vi "find closest point.vi"(11 "Path Data":T1={"Path"=[], "Target Velocities"=[], "Robot Location"=[], "Relative Robot Angle (rad)"=0.0, "Curvature"=0.0, "Lookahead Point"=[3064.399009129367, 18229.833030071386], "Lookahead Index"=8.422809037111724, "Closest Point"=[], "Closest Point Index"=0, "Left Velocity"=0.0, "Right Velocity"=0.0, "Left Encoder Vel"=0, "Right Encoder Vel"=0, "Left Encoder Pos"=0, "Right Encoder Pos"=0, "Inital Robot Angle (deg)"=0.0}) -> (3 "Path Data":T1={"Path"=[], "Target Velocities"=[], "Robot Location"=[], "Relative Robot Angle (rad)"=0.0, "Curvature"=0.0, "Lookahead Point"=[3064.399009129367, 18229.833030071386], "Lookahead Index"=8.422809037111724, "Closest Point"=[], "Closest Point Index"=0, "Left Velocity"=0.0, "Right Velocity"=0.0, "Left Encoder Vel"=0, "Right Encoder Vel"=0, "Left Encoder Pos"=0, "Right Encoder Pos"=0, "Inital Robot Angle (deg)"=0.0})   [LabVIEW 2018]
uses:
  path data.ctl
panel:
  out "Closest Point Index":i32
  out "Closest Point":dbl[](array[numeric])
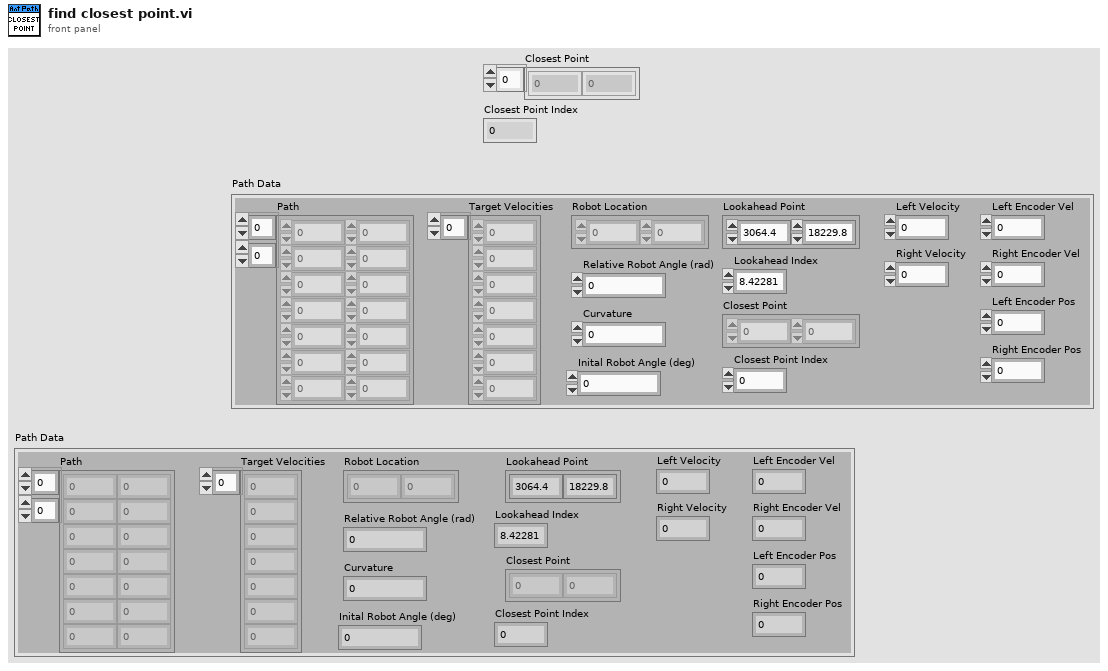
[diagram p1: front panel]
types:
  T1 = typedef "path data.ctl" = cluster{"Path":dbl[][], "Target Velocities":dbl[], "Robot Location":dbl[], "Relative Robot Angle (rad)":dbl, "Curvature":dbl, "Lookahead Point":dbl[], "Lookahead Index":dbl, "Closest Point":dbl[], "Closest Point Index":i32, "Left Velocity":dbl, "Right Velocity":dbl, "Left Encoder Vel":i32, "Right Encoder Vel":i32, "Left Encoder Pos":i32, "Right Encoder Pos":i32, "Inital Robot Angle (deg)":dbl}
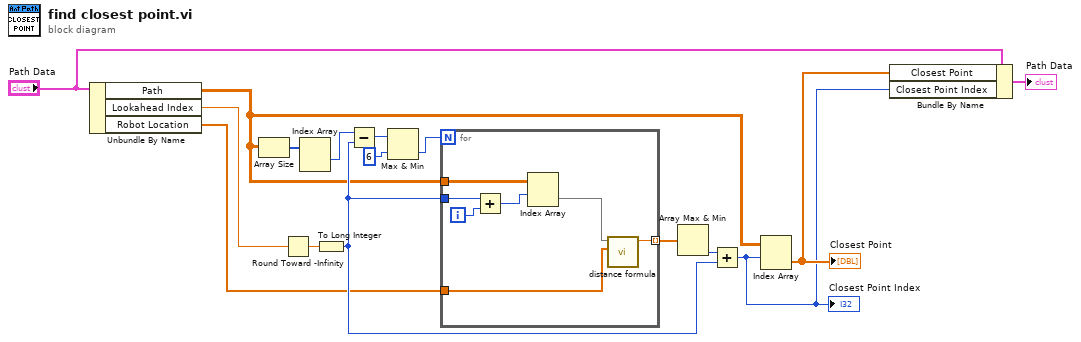
[diagram p0: block diagram]
diagram:
  n1 = Unbundle By Name("Path Data") -> ("Path"=w3:dbl[][], "Lookahead Index"=w2:dbl, "Robot Location"=w1:dbl[])
  n2 = Array Size(array=w3) -> (size(s)=w16:i32[])
  n3 = Round Toward -Infinity(1:w2) -> (0:w14:dbl)
  n4 = Index Array(array=w16) -> (element #1=w15:i32)  [unwired: 2 in, 1 out]
  n5 = To Long Integer(number=w14) -> (32bit integer=w11:i32)
  n6 = Subtract(x=w15, y=w11) -> (x-y=w10:i32)
  n7 = Max & Min(x=w10, y=6) -> (min(x,y)=w8:i32)  [unwired: 1 out]
  n8 = for {
    N: w8 -> [_]
    tunnel: w3 -> [w23]
    tunnel: w11 -> [w20]
    tunnel: w1 -> [w18]
    tunnel: [w17] -> w13 mode=indexing
    i -> [w22]
    n9 = Add(x=w20, y=w22) -> (x+y=w21:i32)
    n10 = Index Array(array=w23, index (row)=w21) -> (element=w19:dbl[])  [unwired: 1 in]
    n11 = call "distance formula.vi"("Point Y"=w18, "Point X"=w19) -> ("Distance"=w17:dbl)  [unwired: 8 in, 1 out]
  }
  n12 = Array Max & Min(array=w13) -> (min index (indices)=w12:i32)  [unwired: 3 out]
  n13 = Add(x=w12, y=w11) -> (x+y=w4:i32)
  "Closest Point Index" <- w4
  n14 = Index Array(array=w3, index (row)=w4) -> (element=w5:dbl[])  [unwired: 1 in]
  "Closest Point" <- w5
  n15 = Bundle By Name(cluster="Path Data", "Closest Point"=w5, "Closest Point Index"=w4) -> (→"Path Data":T1)
